vi "Initialize SUT.vi"(8 "error in (no error)":errorcluster, 11 "XML Report Test in":refnum<class "XML Report Test.lvclass">) -> (0 "error out":errorcluster, 3 "XML Report out":refnum<class "XML Report.lvclass">)   [LabVIEW 2020, in "XML Report Test.lvclass"]
uses:
  XML Report Test.lvclass
  XML Report Test.lvclass/XML Report Test.ctl
  source/Plugins/XML Report/XML Report.lvclass
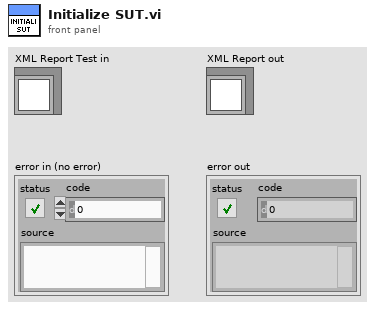
[diagram p1: front panel]
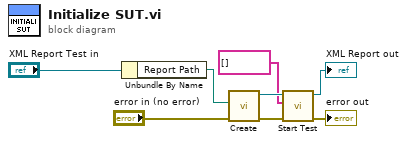
[diagram p0: block diagram]
diagram:
  n1 = Unbundle By Name("XML Report Test in") -> ("Report Path"=w8:path)
  n2 = call "Create.vi"("error in (no error)"="error in (no error)", "Report Path"=w8) -> ("error out"=w6:errorcluster, "XML Report"=w7:refnum<class "XML Report.lvclass">)  [unwired: 8 in]
  n3 = call-dynamic "Start Test.vi"("error in (no error)"=w6, "Tests"=string[] [], "XML Report In"=w7) -> ("error out"=→"error out":errorcluster, "XML Report Out"=→"XML Report out":refnum<class "XML Report.lvclass">)  [unwired: 7 in]
